vi "_Save Users to File.vi"(8 "Error in":errorcluster caption="Error in (no error)", 11 "Array":T1[](array[typedef])) -> (0 "Error out":errorcluster)   [LabVIEW 2020]
uses:
  User-Info.ctl
  User-Role.ctl
  4703436d-49e6-4ed7-825b-d682e24a79d8.vi
  <userlib>/NEVSTOP-Programming-Palette/Configuration/ClusterCfgTable/Flatten Cluster To CfgTable(with DataName).vi
  <userlib>/NEVSTOP-Programming-Palette/Configuration/Ini/ini_configuration_nevstop.lvlib
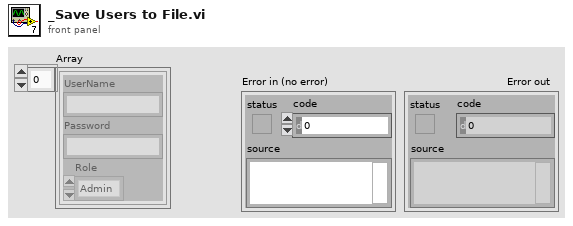
[diagram p1: front panel]
types:
  T1 = typedef "User-Info.ctl" = cluster{"UserName":string, "Password":string, "Role":T2}
  T2 = typedef "User-Role.ctl" = enum16{"Admin", "Engineer", "Operator"}
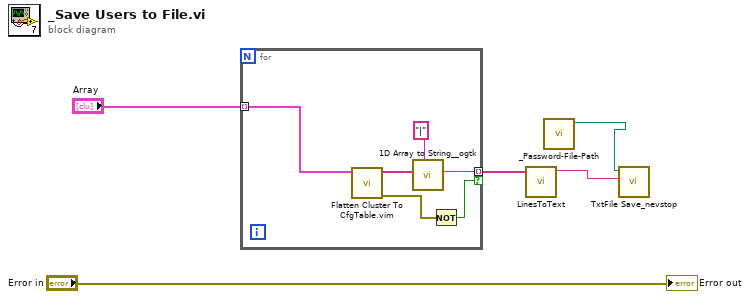
[diagram p0: block diagram]
diagram:
  n1 = for {
    tunnel: [w7] -> w3 mode=indexing if=w9
    tunnel: "Array" -> [w8] mode=indexing
    n2 = call "Flatten Cluster To CfgTable.vim"("Cluster Configuration Typedef"=w8) -> ("error out"=w10:errorcluster, "CfgTable Row"=w11:string[])  [unwired: 8 in, 1 out]
    n3 = call <userlib>:"1D Array to String__ogtk.vi"("delimiter (Tab)"="|", "Array of Strings"=w11) -> ("delimited string"=w7:string)  [unwired: 9 in]
    n4 = Not(x=w10) -> (.not. x?=w9:bool)
  }
  n5 = call <userlib>:"LinesToText.vi"("Lines"=w3) -> ("string"=w1:string)  [unwired: 9 in, 1 out]
  n6 = call "_Password-File-Path.vi"() -> ("Matched Config File"=w2:path)  [unwired: 11 in]
  n7 = call <userlib>:"TxtFile Save_nevstop.vi"("text"=w1, "Path"=w2) -> ()  [unwired: 9 in, 1 out]
  "Error out" <- "Error in"
